vi "UHR-Fleezers Control (fpga) - 10.4.vi"() -> ()   [LabVIEW 2014]
doc: "UHR-Fleezers Instrument Control Code (fpga)"
uses:
  <vilib>/eio/EIONode/EIONode.xnode
  <vilib>/eio/EIOMethodNode/EIOMethodNode.xnode
  <vilib>/rvi/DataTransferAndStorage/Container/XNode/niFpgaContainer.xnode
  <vilib>/Platform/TimedLoop/XDataNode/XDataNode.xnode
  <vilib>/Platform/TimedLoop/XDataNode/nitl_modes.ctl
  <vilib>/Platform/TimedLoop/XDataNode/XDNodeRunTimeDep.lvlib
  <vilib>/Platform/TimedLoop/XDataNode/wakeup.ctl
  <vilib>/Platform/TimedLoop/XDataNode/timing_clust.ctl
  <vilib>/addons/control/pid/fpga.llb/XNode/niFpgaPID.xnode
  <vilib>/rvi/eio/common/nirviEmuTemplateMethod_errors.vi
  <vilib>/rvi/interface/RandomDataEmulation/nirviRandomDataFpgaReadWriteTemplate.vi
panel:
  in  "Connector0/AO6":i16
  in  "Tab Control":T1(tab)=enum."Force FB"
  in  "Trap Pos to FIFO":bool
  in  "AI1 Sets to FIFO":T2={"Set 1"=TRUE, "Set 2"=TRUE, "Set 3"=FALSE}
  in  "N of AI1 Int Acq Sets":i16=2 min=1 max=3 step=1
  out "AI Late Counter":u16
  in  "ai count":u32=400
  out "AI late?":bool
  in  "+ phase":bool
  in  "Phase count adjustment":i16
  out "Relative phase":i16
  in  "AI to FIFO":bool
  out "BD1 Frequency Out 1":u64
  out "BD1 Frequency Out 2":u64
  out "Trap Pos FIFO Timeout":u16
  out "Trap AI FIFO Timeout":u16
  in  "Trap FIFO Set Timeout":i32
  in  "Tab Control 2":T3(tab)
  in  "Swap F1 and F2":bool
  in  "Freq or Amp switch first":bool=TRUE
  in  "Cont. Scan":bool
  in  "Abort scan":bool
  in  "Cycles per step":u64
  in  "Scan BD":bool
  in  "Number of scans":u16
  in  "Scan steps":u64
  in  "Scan freq.  increment":i64
  out "Scanning":bool
  in  "Start scan":bool
  in  "OSK Bd 1":bool
  in  "Reset Bd 1":bool
  in  "RD":bool
  in  "PMODE":bool
  in  "OSK Bd 2":bool
  in  "Reset Bd 2":bool
  in  "Direct RF Box \nCommunication":bool
  in  "Data BD 2":u8 format="%08b"
  in  "Data BD 1":u8 format="%08b"
  in  "Address":u8 format="%02x"
  in  "Update Data":bool
  in  "FPGA Controls\n RF Box":bool
  in  "Number Interlace Cycles":u8=2 min=1 max=3
  in  "Interlace Off Parameters":u8=1 min=1 max=3
  in  "Interlace ON/OFF":bool
  out "DIO Relative phase":i16
  in  "Phase count adjustment (DIO)":i16
  in  "+ phase (DIO)":bool
  out "DIO Late Counter":u16
  out "DIO Late?":bool
  in  "DIO count 1 (ticks)":u32=400
  in  "DIO count 2 (ticks)":u32=400
  in  "DIO count 3 (ticks)":u32=400
  out "AI2 Y Sum Set 2":i16
  out "AI2 Y Sum Set 1":i16
  in  "FB Gains Set 1":T4={"proportional gain (Kc)"=10, "integral gain (Kc*Ts/Ti)"=5, "derivative gain (Kc*Td/Ts)"=0}
  in  "FB Setpoint Set 1":i16 min=0 step=1
  in  "FB Reset Set 1":bool
  in  "FB On/Off Set 1":bool
  in  "FB Reset Set 2":bool
  in  "FB On/Off Set 2":bool
  in  "FB Setpoint Set 2":i16 min=0 step=1
  in  "FB Gains Set 2":T4={"proportional gain (Kc)"=10, "integral gain (Kc*Ts/Ti)"=5, "derivative gain (Kc*Td/Ts)"=0}
  in  "FB output range 2":cluster{"output high":i16, "output low":i16}={"output high"=3000, "output low"=0}
  in  "FB output range 1":cluster{"output high":i16, "output low":i16}={"output high"=3000, "output low"=0}
  out "Scan I":u64
  in  "Amp switch delay":u16=5
  in  "Freq switch delay":u16
  in  "BD 2 Amplitude 1":u16
  in  "BD 1 Amplitude 1":u16
  in  "BD 2 Frequency 1":u64
  in  "BD 1 Frequency 1":u64
  in  "BD 2 Amplitude 2":u16
  in  "BD 1 Amplitude 2":u16
  in  "BD 2 Frequency 2":u64
  in  "BD 1 Frequency 2":u64
  in  "BD 2 Amplitude 3":u16
  in  "BD 1 Amplitude 3":u16
  in  "BD 2 Frequency 3":u64
  in  "BD 1 Frequency 3":u64
  in  "Negate Diff?":bool
  in  "Diff FB Measurement?":bool
  in  "FB Trig Integrate":u32=1
  out "TTrig?":bool
  in  "TTrig Negate Pos":bool=TRUE
  out "Trap Pos FB Int Signal":fxp<+/-,24,9> format="%.18g"
  out "Trap Pos FB Int-Norm Signal":fxp<+/-,16,1> format="%.16g"
  in  "FPGA TTrig Thresh":i64
  in  "FPGA Trap Trig":bool
  out "Trap Pos FB Action":i64
  in  "Trap Pos. FB Offset Factor":i64
  in  "Trap Pos. FB Mult Factor":i64=2
  in  "Trap Pos. FB Range":T5={"output high"=0.999969482421875, "output low"=-1.0}
  in  "Trap Pos. FB Gains":T6={"proportional gain (Kc)"=0.0, "integral gain (Kc*Ts/Ti)"=10.0, "derivative gain (Kc*Td/Ts)"=0.0} {"proportional gain (Kc)" format="%.11g"; "integral gain (Kc*Ts/Ti)" format="%.11g"; "derivative gain (Kc*Td/Ts)" format="%.11g"}
  in  "Trap Pos. FB Reset":bool
  in  "Trap Pos FB Monitor T1 or T2":bool
  in  "AI1 X Scale":u16
  in  "Trap Pos FB Int Count":u16=100
  in  "Trap Pos FB Negate Action":bool
  out "AI1 X Set 2":fxp<+/-,16,1>
  out "AI1 X Set 1":fxp<+/-,16,1>
  in  "Trap Pos. FB SP":fxp<+/-,16,1>
  in  "Force feedback":bool
  out "TTrig Sig":i64
  out "TTrig Fin Thresh":i64
  out "Numeric":i32
  out "AO2 2":i16
  out "AO1 2":i16
  in  "1D or 2D Scan?":bool
  in  "Abort scan (MCL)":bool
  in  "MCL Scan Axis":bool
  in  "Cont. Scan (MCL)":bool
  out "Scan I (MCL)":u64
  in  "Number of scans (MCL)":u16
  out "Scanning MCL":bool
  in  "Scan steps (MCL)":u64
  in  "Cycles per step (MCL)":u64
  in  "Scan freq.  increment (MCL)":i16
  in  "Start scan (MCL)":bool
  in  "AO2":i16
  in  "AO1":i16
  out "MCL Late Counter":u16
  out "MCL Late?":bool
  in  "MCL count":u32=800
  out "MCL Relative Phase":i16
  in  "Phase count adjustment (MCL)":i16
  in  "+ phase (MCL)":bool
  in  "APD Gate Operating Mode":u8 max=2 step=1
  in  "Invert APD Gate":bool
  in  "APD Gate OFF Count":u32=100
  in  "APD Gate ON Count":u32=300
  out "APD 1 Gate Late Counter":u16
  out "APD 1 Gate Late?":bool
  out "APD 1 Gate Relative Phase":i16
  in  "Phase count adjustment (APD 1 Gate)":i16
  in  "+ phase (APD 1 Gate)":bool
  out "APD 2 Counts 0":u32
  out "APD 2 Counts 1":u32
  out "APD 1 Counts 0":u32
  out "APD 1 Counts 1":u32
  out "APD1 out state":bool
  in  "APD 2 AO scale factor":i16=1
  in  "APD 1 AO scale factor":i16=1
  in  "APD to FIFO":bool
  in  "APD Acq Rate Count":u32=20000000
  out "APD Acq Late Counter":u16
  out "APD Acq Late?":bool
  out "APD Acq Relative Phase":i16
  in  "Phase Count Adjustment (APD Acq)":i16
  in  "+ phase (APD Acq)":bool
  in  "Phase count adjustment (APD 2 Gate)":i16
  out "APD 2 Gate Late Counter":u16
  out "APD 2 Gate Late?":bool
  out "APD 2 Gate Relative Phase":i16
  in  "+ phase (APD 2 Gate)":bool
  out "APD2 out state":bool
  in  "Green Filter Flipper":bool
  out "Green FB Signals":T7
  in  "Green FB Count":u32=1200
  out "Green Late Counter":u16
  out "Green FB Late?":bool
  out "Green FB Relative Phase":i16
  in  "Phase count adjustment (Green FB)":i16=10
  in  "+ phase (Green FB)":bool
  out "Green FB Sum":i16
  in  "Green int current ON count adj":u32=150
  in  "Current Out":u16=30000
  in  "Green FB On/Off":bool
  in  "Green FB Setpoint":i16=250 min=0 step=1
  in  "Green FB Gains":T4={"proportional gain (Kc)"=10, "integral gain (Kc*Ts/Ti)"=5, "derivative gain (Kc*Td/Ts)"=0}
  in  "Green FB Reset":bool
  in  "Operating Mode 2":u8=2 max=2 step=1
  in  "Invert GI 2":bool
  in  "Green interlace OFF count 2":u32=900
  in  "Green interlace ON count 2":u32=300
  out "GI Late Counter 2":u16
  out "GI Late? 2":bool
  out "GI Relative phase 2":i16
  in  "Phase count adjustment (GI) 2":i16=20
  in  "+ phase (GI) 2":bool
  in  "Green interlace OFF count":u32=100
  out "GI Relative phase":i16
  in  "Phase count adjustment (GI)":i16
  in  "+ phase (GI)":bool
  out "GI Late?":bool
  in  "Green interlace ON count":u32=300
  out "GI Late Counter":u16
  in  "Invert GI":bool
  in  "Operating Mode":u8 max=2 step=1
  in  "Chassis2/Mod4/AO1":u16
  # "Only one of these can be on\nat a time:"
  # "Raster Scan AOD"
  # "1 (X)"
  # "2 (Y)"
  # "IR Intensity Feedback (RF BD 1)"
  # "FB Triggering Excitation Laser"
  # "AO1 (Y)"
  # "2D"
  # "1D"
  # "AO2 (X)"
  # "APD AO for aligning"
  # "Detection Loop"
  # "Green fluorescent laser digital gate interlacing loop"
  # "0 Forced ON\n1 Forced OFF\n2 Interlacing"
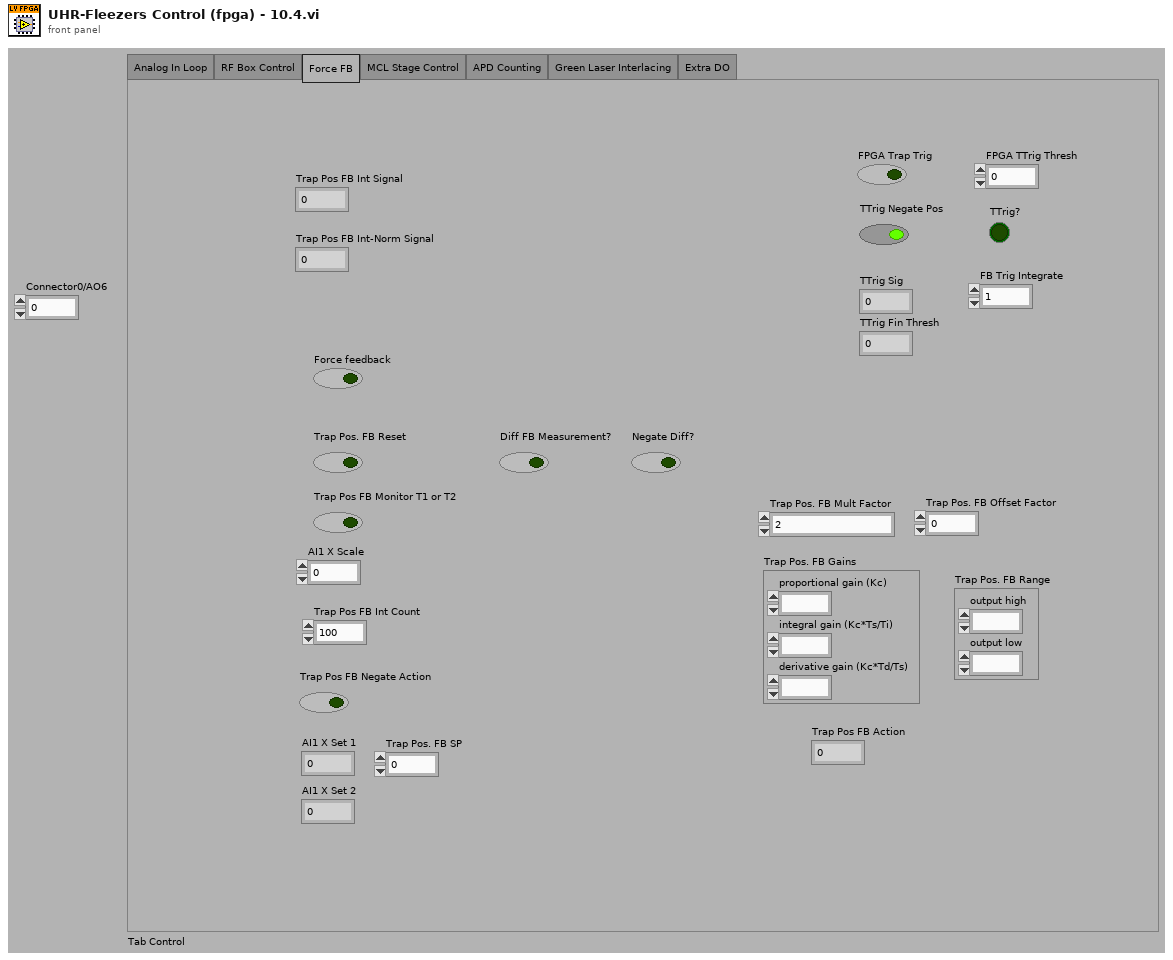
[diagram p1: front panel]
types:
  T1 = enum32{"Analog In Loop", "RF Box Control", "Force FB", "MCL Stage Control", "APD Counting", "Green Laser Interlacing", "Extra DO"}
  T2 = cluster{"Set 1":bool, "Set 2":bool, "Set 3":bool}
  T3 = enum32{"Controls", "Interlacing Frequency and Amplitude Values"}
  T4 = cluster{"proportional gain (Kc)":i16, "integral gain (Kc*Ts/Ti)":i16, "derivative gain (Kc*Td/Ts)":i16}
  T5 = cluster{"output high":fxp<+/-,16,1>, "output low":fxp<+/-,16,1>}
  T6 = cluster{"proportional gain (Kc)":fxp<+/-,16,8>, "integral gain (Kc*Ts/Ti)":fxp<+/-,16,8>, "derivative gain (Kc*Td/Ts)":fxp<+/-,16,8>}
  T7 = cluster{"Green FB Ch 0":i16, "Green FB Ch 1":i16, "Green FB Ch 2":i16}
  T8 = typedef "XDNodeRunTimeDep.lvlib/timing_clust.ctl" = cluster{"Expected End [f-1]":u64, "Actual End [f-1]":u64, "Finished Late? [f-1]":bool, "Expected End [i-1]":u64, "Actual End [i-1]":u64, "Finished Late? [i-1]":bool, "Expected Start [i]":u64, "Actual Start [i]":u64, "Expected Start [f]":u64, "Actual Start [f]":u64, "Source Name":string, "Structure Name":string, "Period":i64, "Deadline":i64, "Offset":i64, "Start":i64, "Priority":i32, "Timeout":i32, "Mode":T9, "Wakeup Reason":T10, "Error":errorcluster, "Source Type":string, "Secondary Source Type":string, "Global End Time":u64, "Global Start Time":u64, "Frame Duration":u64, "Iteration Duration":u64, "Assigned CPU":i32, "I/O Scan Engine Mode":u32}
  T9 = typedef "XDNodeRunTimeDep.lvlib/nitl_modes.ctl" = enum32{"No Change", "Process missed periods, maintain original phase", "Discard missed periods, maintain original phase", "Process missed periods, ignore original phase", "Discard missed periods, ignore original phase"}
  T10 = typedef "XDNodeRunTimeDep.lvlib/wakeup.ctl" = enum32{"Normal", "Aborted", "Asynchronous wakeup", "Timing source error", "Timed loop error", "Timeout"}
  T11 = cluster{"Chassis2/Mod1/AI0":void, "Chassis2/Mod1/AI1":void, "Chassis2/Mod1/AI2":void}
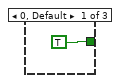
[diagram p2: hidden frame]
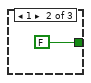
[diagram p3: hidden frame]
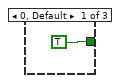
[diagram p5: hidden frame]
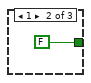
[diagram p6: hidden frame]
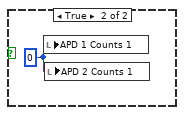
[diagram p7: hidden frame]
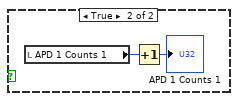
[diagram p9: hidden frame]
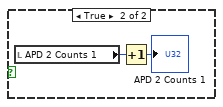
[diagram p10: hidden frame]
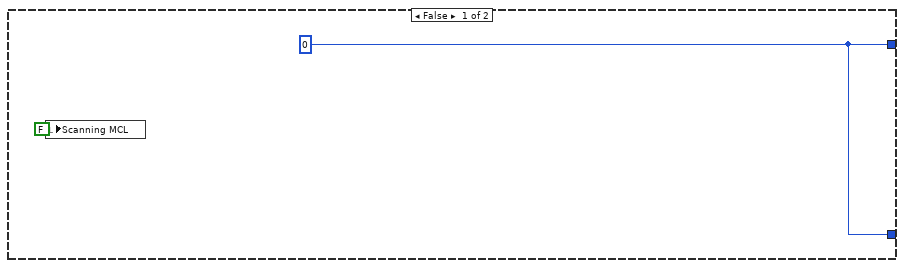
[diagram p11: hidden frame]
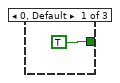
[diagram p12: hidden frame]
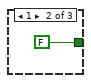
[diagram p13: hidden frame]
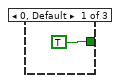
[diagram p14: hidden frame]
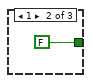
[diagram p15: hidden frame]
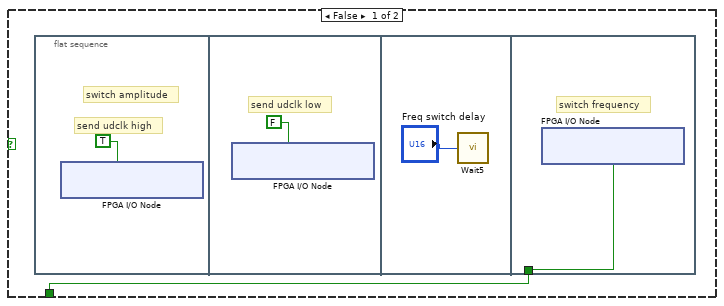
[diagram p18: hidden frame]
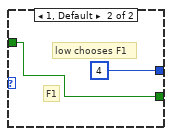
[diagram p20: hidden frame]
diagram:
  w3 = FALSE
  # "timing array current index"
  # "timing array"
  # "timing counter (phase adjusted here)"
  # "late counter"
  n1 = flat-sequence "FPGA initialization to do before running any of the loops" {
    tunnel: [u32 0 ("DIO count 3 (ticks)")] -> w2
    tunnel: [w10] -> _
    frame #0 {
      # "Start up expansion chassis early\nto avoid delays later"
      # "This pin controls udclk on the RF boards.\nWhen initially configuring the boards, this pin needs to be\nconfigured as a high impedance input.  Later it will be switched\nto an output."
      # "Initial setting of DIO data and \naddress to low (before reset).  \nThis needs to happen before the other\ncontrol method loops execute."
      n2 = xnode "FPGA I/O Node"("Chassis2/Mod4/AO0"=u16 0) -> ("Chassis2/Mod1/AI0"=w10)  [unwired: 2 in, 2 out]
      n3 = xnode "FPGA I/O Method Node"("Enable"=FALSE) -> ()  [unwired: 1 in, 1 out]
      n4 = xnode "FPGA I/O Node"("Connector1/DIO0"=FALSE, "Connector1/DIO1"=FALSE, "Connector1/DIO2"=FALSE, "Connector1/DIO3"=FALSE, "Connector1/DIO4"=FALSE, "Connector1/DIO5"=FALSE, "Connector1/DIO6"=FALSE, "Connector1/DIO7"=FALSE, "Connector1/DIO8"=FALSE, "Connector1/DIO9"=FALSE, "Connector1/DIO10"=FALSE, "Connector1/DIO11"=FALSE, "Connector1/DIO12"=FALSE, "Connector1/DIO13"=FALSE, "Connector1/DIO15"=FALSE, "Connector1/DIO20"=FALSE, "Connector1/DIO21"=FALSE, "Connector1/DIO22"=FALSE, "Connector1/DIO23"=FALSE, "Connector1/DIO24"=FALSE, "Connector1/DIO25"=FALSE, "Connector1/DIO26"=FALSE, "Connector1/DIO27"=FALSE, "Connector1/DIO14"=FALSE) -> ()  [unwired: 24 in, 24 out]
    }
  }
  n5 = local read "AO1"() -> (w7:i16)
  n6 = local read "AO2"() -> (w6:i16)
  n7 = node-c288() -> (w5:T8)  [unwired: 1 in]
  n8 = while "APD 1 Counter" {
    tunnel: w2 -> [_]
    stop <- FALSE stop-if-true
    n9 = flat-sequence {
      frame #0 {
        n10 = xnode "FPGA I/O Method Node"("FPGA I/O In"=refnum<k21> "Connector0/DIO0" ("APD 1 DO"), "Timeout"=-1) -> ()  [unwired: 2 out]
      }
      frame #1 {
        n11 = local read "APD1 out state"() -> (w41:bool)
        n12 = case shown="False" w41 {
          frame False {
            n13 = local read "APD 1 Counts 0"() -> (w43:u32)
            n14 = Increment(x=w43) -> (x+1=→"APD 1 Counts 0":u32)
          }
          frame True {
            n15 = local read "APD 1 Counts 1"() -> (w45:u32)
            n16 = Increment(x=w45) -> (x+1=→"APD 1 Counts 1":u32)
          }
        }
      }
    }
  }
  n17 = while "APD 2 Counter" {
    tunnel: w2 -> [_]
    stop <- FALSE stop-if-true
    n18 = flat-sequence {
      frame #0 {
        n19 = xnode "FPGA I/O Method Node"("FPGA I/O In"=refnum<k21> "Connector0/DIO1" ("APD 2 DO"), "Timeout"=-1) -> ()  [unwired: 2 out]
      }
      frame #1 {
        n20 = local read "APD2 out state"() -> (w49:bool)
        n21 = case shown="False" w49 {
          frame False {
            n22 = local read "APD 2 Counts 0"() -> (w51:u32)
            n23 = Increment(x=w51) -> (x+1=→"APD 2 Counts 0":u32)
          }
          frame True {
            n24 = local read "APD 2 Counts 1"() -> (w53:u32)
            n25 = Increment(x=w53) -> (x+1=→"APD 2 Counts 1":u32)
          }
        }
      }
    }
  }
  n26 = while "APD 2 Gating" {
    shift-right: [w57] -> _
    shift-left: w2 -> [w62]
    shift-right: [w56] -> _
    shift-left: w3 -> [w54]
    stop <- FALSE stop-if-true
    n27 = flat-sequence {
      tunnel: w62 -> [w65]
      tunnel: [w66] -> w60
      tunnel: [w65] -> w58
      tunnel: [w64] -> w55
      tunnel: w54 -> [w64]
      tunnel: [w69] -> w61
      tunnel: w60 -> [w69]
      tunnel: [w68] -> w59
      tunnel: w58 -> [w68]
      tunnel: w55 -> [w67]
      tunnel: [w87] -> w57
      tunnel: w61 -> [w98]
      tunnel: w59 -> [w96]
      tunnel: [w91] -> w56
      frame #0 {
        n28 = call "Loop Timer8"("Count(Ticks)"=w65) -> ("Tick Count(Ticks)"=w66:u32)
      }
      frame #1 {
        # "(need 4 channels/APD)"
        n29 = xnode "FPGA I/O Node"("Connector0/DIO8"=w67, "Connector0/DIO9"=w67, "Connector0/DIO10"=w67, "Connector0/DIO11"=w67) -> ()  [unwired: 4 in, 4 out]
      }
      frame #2 {
        n30 = local read "APD Gate ON Count"() -> (w80:u32)
        n31 = local read "APD Gate OFF Count"() -> (w79:u32)
        n32 = feedback #1(TRUE) -> (w93:bool)
        n33 = feedback-in #2(w98) -> ()
        n34 = feedback #2(w98) -> (w81:u32)
        n35 = Not(x=w93) -> (.not. x?=w90:bool)
        n36 = feedback-in #1(w90) -> ()
        n37 = Subtract(x=w98, y=w81) -> (x-y=w97:u32)
        n38 = Select(t=w80, s=w90, f=w79) -> (s? t:f=w95:u32)
        n39 = Subtract(x=w97, y=w96) -> (x-y=w72:u32)
        n40 = Subtract(x=w95, y=w72) -> (x-y=w86:u32)
        n41 = Number To Boolean Array(number=w72) -> (Boolean array=w71:bool[])
        n42 = Or Array Elements(Boolean array=w71) -> (logical OR=w70:bool)
        "APD 2 Gate Late?" <- w70
        n43 = Boolean To (0,1)(Boolean="+ phase (APD 2 Gate)") -> (0, 1=w84:i16)
        n44 = Multiply(x=w84, y="Phase count adjustment (APD 2 Gate)") -> (x*y=w82:i16)
        n45 = Boolean To (0,1)(Boolean=w70) -> (0, 1=w77:i16)
        n46 = Add(x=w86, y=w82) -> (x+y=w87:u32)
        n47 = To Unsigned Word Integer(number=w77) -> (unsigned 16bit integer=w74:u16)
        n48 = feedback #3(i16 0) -> (w89:i16)
        n49 = Subtract(x=w89, y=w82) -> (x-y=w88:i16)
        "APD 2 Gate Relative Phase" <- w88
        n50 = feedback-in #3(w88) -> ()
        n51 = feedback #4(u16 0) -> (w75:u16)
        n52 = Add(x=w74, y=w75) -> (x+y=w73:u16)
        "APD 2 Gate Late Counter" <- w73
        n53 = feedback-in #4(w73) -> ()
        n54 = local read "APD Gate Operating Mode"() -> (w78:u8)
        n55 = case shown="2" w78 {
          tunnel: [TRUE FALSE w104] -> w91
          tunnel: w93 -> [_ _ w102]
          frame 0, Default {
          }
          frame 1 {
          }
          frame 2 {
            n56 = local read "Invert APD Gate"() -> (w101:bool)
            n57 = Not(x=w102) -> (.not. x?=w103:bool)
            n58 = Select(t=w103, s=w101, f=w102) -> (s? t:f=w104:bool)
          }
        }
      }
    }
  }
  n59 = while "DAQ AI set 1" {
    shift-right: [w105] -> _
    shift-left: w2 -> [w110]
    stop <- FALSE stop-if-true
    n60 = flat-sequence {
      tunnel: w110 -> [w120]
      tunnel: [w121] -> w108
      tunnel: [w120] -> w107
      tunnel: [w131] -> w118
      tunnel: [w130] -> w117
      tunnel: [w129] -> w116
      tunnel: [w128] -> w115
      tunnel: [w127] -> w114
      tunnel: [w126] -> w113
      tunnel: [w125] -> w112
      tunnel: [w124] -> w111
      tunnel: [w123] -> w109
      tunnel: w108 -> [w123]
      tunnel: w107 -> [w122]
      tunnel: [w122] -> w106
      tunnel: [w160] -> w105
      tunnel: w118 -> [w188]
      tunnel: w117 -> [w152]
      tunnel: w116 -> [w153]
      tunnel: w115 -> [w187]
      tunnel: w114 -> [w176]
      tunnel: w113 -> [w175]
      tunnel: w112 -> [w174]
      tunnel: w111 -> [w173]
      tunnel: w109 -> [w170]
      tunnel: w106 -> [w167]
      frame #0 {
        n61 = call "Loop Timer3"("Count(Ticks)"=w120) -> ("Tick Count(Ticks)"=w121:u32)
      }
      frame #1 {
        n62 = xnode "FPGA I/O Node"("Connector1/DIO31"=TRUE ("Connector1/DIO33")) -> ("Connector0/AI0"=w131, "Connector0/AI1"=w130, "Connector0/AI2"=w129, "Connector0/AI3"=w128, "Connector0/AI4"=w127, "Connector0/AI5"=w126, "Connector0/AI6"=w125, "Connector0/AI7"=w124)  [unwired: 9 in, 9 out]
      }
      frame #2 {
        w156 = FALSE ("AI to FIFO")
        # "Adjust phase after data acquired if button pressed"
        n63 = feedback #5(i16 1) -> (w180:i16)
        n64 = Increment(x=w180) -> (x+1=w186:i16)
        n65 = Scale By Power Of 2(n="AI1 X Scale", x=w152) -> (x*2^n=w150:dbl)
        n66 = Greater?(x=w186, y="N of AI1 Int Acq Sets") -> (0:w183:bool)
        n67 = Select(t=i16 1, s=w183, f=w186) -> (s? t:f=w185:i16)
        n68 = feedback-in #5(w185) -> ()
        n69 = Divide(x=w150, y=w153) -> (x/y=w149:fxp<+/-,16,1>)
        n70 = feedback #6(w156) -> (w154:bool)
        n71 = feedback #7(w156) -> (w172:bool)
        n72 = case shown="1, Default" w180 {
          tunnel: w153 -> [w210 w218 _]
          tunnel: "AI1 Sets to FIFO" -> [w214 w222 w228]
          tunnel: [w213 w221 w227] -> w177
          tunnel: ["AI to FIFO" w220 w226] -> w171
          tunnel: w172 -> [_ w220 w226]
          tunnel: ["Trap Pos to FIFO" w219 w225] -> w155
          tunnel: w154 -> [_ w219 w225]
          tunnel: w149 -> [w209 w217 _]
          tunnel: [w208 w215 FALSE] -> w136
          tunnel: [w207 w216 u64 0 ("BD1 Frequency Out 2")] -> w135
          frame 1, Default {
            n73 = Unbundle By Name(w214) -> ("Set 1"=w213:bool)
            n74 = local read "BD1 Frequency Out 1"() -> (w207:u64)
            n75 = Compound Arithmetic op=AND("Trap Pos to FIFO", w213, "AI to FIFO") -> (w208:bool)
            "AI2 Y Sum Set 1" <- w210
            "AI1 X Set 1" <- w209
          }
          frame 2 {
            n76 = Unbundle By Name(w222) -> ("Set 2"=w221:bool)
            n77 = local read "BD1 Frequency Out 2"() -> (w216:u64)
            n78 = Compound Arithmetic op=AND(w219, w221, w220) -> (w215:bool)
            "AI2 Y Sum Set 2" <- w218
            "AI1 X Set 2" <- w217
          }
          frame 3 {
            n79 = Unbundle By Name(w228) -> ("Set 3"=w227:bool)
          }
        }
        n80 = And(x=w177, y=w171) -> (x .and. y?=w179:bool)
        n81 = case shown="True" w179 {
          tunnel: w188 -> [_ w242]
          tunnel: w152 -> [_ w241]
          tunnel: w153 -> [_ w240]
          tunnel: w187 -> [_ w239]
          tunnel: w176 -> [_ w238]
          tunnel: w175 -> [_ w237]
          tunnel: w174 -> [_ w236]
          tunnel: w173 -> [_ w235]
          tunnel: 0 ("DMA buffer timeout") -> [_ w244]
          frame False {
          }
          frame True {
            n82 = Build Array(w242, w241, w240, w239, w238, w237, w236, w235) -> (w243:void[])
            n83 = for {
              tunnel: w243 -> [w246] mode=indexing
              tunnel: w244 -> [w247]
              tunnel: [w245] -> w233 mode=indexing
              n84 = xnode ("FIFO Write")("Element"=w246, "Timeout"=w247) -> ("Timed Out?"=w245:bool)  [unwired: 1 in, 1 out]
            }
            n85 = Or Array Elements(Boolean array=w233) -> (logical OR=w230:bool)
            n86 = Boolean To (0,1)(Boolean=w230) -> (0, 1=w232:i16)
            n87 = feedback #8(u16 0) -> (w231:u16)
            n88 = Add(x=w232, y=w231) -> (x+y=w229:u16)
            "Trap AI FIFO Timeout" <- w229
            n89 = feedback-in #8(w229) -> ()
          }
        }
        n90 = feedback-in #6(w155) -> ()
        n91 = feedback-in #7(w171) -> ()
        n92 = case shown="True" w136 {
          tunnel: w135 -> [_ w194]
          tunnel: [u8 0 w191] -> w134
          frame False {
          }
          frame True {
            n93 = Split Number(x=w194) -> (hi(x)=w195:u32, lo(x)=w196:u32)
            n94 = Split Number(x=w195) -> (lo(x)=w197:u16)  [unwired: 1 out]
            n95 = Split Number(x=w196) -> (hi(x)=w198:u16, lo(x)=w199:u16)
            n96 = Build Array "BD 1 nu Stack"(w197, w198, w199) -> (w193:u16[])
            n97 = for {
              tunnel: w193 -> [w206] mode=indexing
              shift-right: [w202] -> w191
              shift-left: u8 0 -> [w203]
              n98 = xnode ("FIFO Method Node")("Element"=w206, "Timeout"="Trap FIFO Set Timeout") -> ("Timed Out?"=w205:bool)  [unwired: 1 in, 1 out]
              n99 = Boolean To (0,1)(Boolean=w205) -> (0, 1=w204:i16)
              n100 = To Unsigned Byte Integer(number=w204) -> (unsigned 8bit integer=w201:u8)
              n101 = Add(x=w201, y=w203) -> (x+y=w202:u8)
            }
          }
        }
        n102 = To Unsigned Word Integer(number=w134) -> (unsigned 16bit integer=w133:u16)
        n103 = feedback #9(u16 0) -> (w147:u16)
        n104 = Add(x=w133, y=w147) -> (x+y=w146:u16)
        "Trap Pos FIFO Timeout" <- w146
        n105 = feedback-in #9(w146) -> ()
        n106 = feedback-in #10(w170) -> ()
        n107 = feedback #10(w170) -> (w169:u32)
        n108 = Subtract(x=w170, y=w169) -> (x-y=w168:u32)
        n109 = xnode "I/O Node"("Connector1/DIO31"=FALSE ("Connector1/DIO34")) -> ()  [unwired: 1 in, 1 out]
        n110 = Subtract(x=w168, y=w167) -> (x-y=w138:u32)
        n111 = Boolean To (0,1)(Boolean="+ phase") -> (0, 1=w163:i16)
        n112 = Multiply(x=w163, y="Phase count adjustment") -> (x*y=w157:i16)
        n113 = Subtract(x="ai count", y=w138) -> (x-y=w161:u32)
        n114 = Number To Boolean Array(number=w138) -> (Boolean array=w139:bool[])
        n115 = feedback #11(i16 0) -> (w159:i16)
        n116 = Add(x=w161, y=w157) -> (x+y=w160:u32)
        n117 = Subtract(x=w159, y=w157) -> (x-y=w158:i16)
        "Relative phase" <- w158
        n118 = feedback-in #11(w158) -> ()
        n119 = Or Array Elements(Boolean array=w139) -> (logical OR=w137:bool)
        "AI late?" <- w137
        n120 = Boolean To (0,1)(Boolean=w137) -> (0, 1=w144:i16)
        n121 = To Unsigned Word Integer(number=w144) -> (unsigned 16bit integer=w141:u16)
        n122 = feedback #12(u16 0) -> (w142:u16)
        n123 = Add(x=w141, y=w142) -> (x+y=w140:u16)
        "AI Late Counter" <- w140
        n124 = feedback-in #12(w140) -> ()
      }
    }
  }
  n125 = while "MCL stage control" {
    shift-right: [w263] -> _
    shift-left: w2 -> [w266]
    shift-right: [w256] -> _
    shift-left: w7 -> [w253]
    shift-right: [w255] -> _
    shift-left: w6 -> [w251]
    i -> [w250]
    stop <- FALSE stop-if-true
    n126 = flat-sequence {
      tunnel: w266 -> [w270]
      tunnel: [w271] -> w262
      tunnel: [w270] -> w260
      tunnel: [w269] -> w254
      tunnel: w253 -> [w269]
      tunnel: [w268] -> w252
      tunnel: w251 -> [w268]
      tunnel: w262 -> [w275]
      tunnel: [w275] -> w261
      tunnel: w260 -> [w274]
      tunnel: [w274] -> w259
      tunnel: w254 -> [w273]
      tunnel: w252 -> [w272]
      tunnel: [w273] -> w249
      tunnel: [w272] -> w248
      tunnel: w261 -> [w285]
      tunnel: w259 -> [w284]
      tunnel: [w285] -> w265
      tunnel: [w284] -> w264
      tunnel: [w283] -> w258
      tunnel: [w282] -> w257
      tunnel: w249 -> [w277]
      tunnel: w248 -> [w276]
      tunnel: [w357] -> w263
      tunnel: w265 -> [w364]
      tunnel: w264 -> [w361]
      tunnel: w258 -> [w359]
      tunnel: w257 -> [w358]
      tunnel: [w359] -> w256
      tunnel: [w358] -> w255
      frame #0 {
        n127 = call "Loop Timer5"("Count(Ticks)"=w270) -> ("Tick Count(Ticks)"=w271:u32)
      }
      frame #1 {
        n128 = xnode "FPGA I/O Node"("Connector0/AO1"=w273, "Connector0/AO2"=w272) -> ()  [unwired: 2 in, 2 out]
      }
      frame #2 {
        n129 = local read "Scanning MCL"() -> (w297:bool)
        n130 = Or(x=w297, y="Start scan (MCL)") -> (x .or. y?=w292:bool)
        n131 = Not(x="Abort scan (MCL)") -> (.not. x?=w290:bool)
        n132 = And(x=w290, y=w292) -> (x .and. y?=w289:bool)
        n133 = case "Raster scan" shown="True" w289 {
          tunnel: [w298 w341] -> w294
          tunnel: "Start scan (MCL)" -> [_ w326]
          tunnel: [w298 w302] -> w278
          frame False {
            w298 = i16 0
            n134 = local write "Scanning MCL"(FALSE ("scanning")) -> ()
          }
          frame True {
            w312 = i16 0
            w311 = u64 0
            # "scan incr."
            # "freq. incr. mult."
            # "count steps"
            # "count number of cycles"
            n135 = feedback #13(w311) -> (w338:u64)
            n136 = Select(t=w311, s=w326, f=w338) -> (s? t:f=w340:u64)
            n137 = Increment(x=w340) -> (x+1=w337:u64)
            n138 = Greater?(x="Cycles per step (MCL)", y=w337) -> (0:w321:bool)
            n139 = Select(t=w337, s=w321, f=w311) -> (s? t:f=w336:u64)
            n140 = feedback-in #13(w336) -> ()
            n141 = feedback #14(w311) -> (w335:u64)
            n142 = Select(t=w311, s=w326, f=w335) -> (s? t:f=w330:u64)
            n143 = Increment(x=w330) -> (x+1=w334:u64)
            n144 = Add(x="Scan steps (MCL)", y="Scan steps (MCL)") -> (x+y=w333:u64)
            n145 = Select(t=w330, s=w321, f=w334) -> (s? t:f=w316:u64)
            n146 = Greater?(x=w333, y=w316) -> (0:w315:bool)
            n147 = Select(t=w316, s=w315, f=w311) -> (s? t:f=w331:u64)
            n148 = feedback-in #14(w331) -> ()
            n149 = Equal?(x="Scan steps (MCL)", y=w316) -> (x = y?=w320:bool)
            n150 = Greater?(x="Scan steps (MCL)", y=w330) -> (0:w329:bool)
            n151 = feedback #15(w312) -> (w332:i16)
            n152 = Select(t=w312, s=w326, f=w332) -> (s? t:f=w318:i16)
            n153 = Increment(x=w318) -> (x+1=w328:i16)
            n154 = Decrement(x=w318) -> (x-1=w327:i16)
            n155 = Select(t=w328, s=w329, f=w327) -> (s? t:f=w319:i16)
            n156 = Select(t=w318, s=w320, f=w319) -> (s? t:f=w317:i16)
            n157 = Select(t=w318, s=w321, f=w317) -> (s? t:f=w313:i16)
            n158 = Select(t=w313, s=w315, f=w312) -> (s? t:f=w314:i16)
            n159 = feedback-in #15(w314) -> ()
            n160 = feedback #16(w311) -> (w325:u64)
            n161 = Select(t=w311, s=w326, f=w325) -> (s? t:f=w300:u64)
            n162 = Increment(x=w300) -> (x+1=w322:u64)
            n163 = Select(t=w300, s=w315, f=w322) -> (s? t:f=w301:u64)
            n164 = Greater?(x="Number of scans (MCL)", y=w301) -> (0:w308:bool)
            n165 = Multiply(x="Scan freq.  increment (MCL)", y=w318) -> (x*y=w341:i16)
            n166 = Select(t=TRUE, s="Cont. Scan (MCL)", f=w308) -> (s? t:f=w307:bool)
            "Scanning MCL" <- w307
            n167 = Select(t=w301, s=w307, f=w311) -> (s? t:f=w323:u64)
            n168 = feedback-in #16(w323) -> ()
            n169 = Increment(x=w301) -> (x+1=→"Scan I (MCL)":u64)
            n170 = To Word Integer(number=w300) -> (16bit integer=w303:i16)
            n171 = Multiply(x=w303, y="Scan freq.  increment (MCL)") -> (x*y=w302:i16)
          }
        }
        n172 = Select(t=w278, s="1D or 2D Scan?", f=i16 0) -> (s? t:f=w279:i16)
        n173 = Select(t=w279, s="MCL Scan Axis", f=w294) -> (s? t:f=w293:i16)
        n174 = Select(t=w294, s="MCL Scan Axis", f=w279) -> (s? t:f=w295:i16)
        n175 = Add(x=w293, y="AO2") -> (x+y=w282:i16)
        n176 = Add(x="AO1", y=w295) -> (x+y=w283:i16)
        "AO1 2" <- w277
        "AO2 2" <- w276
      }
      frame #3 {
        n177 = feedback-in #17(w364) -> ()
        n178 = feedback #17(w364) -> (w363:u32)
        n179 = Boolean To (0,1)(Boolean="+ phase (MCL)") -> (0, 1=w355:i16)
        n180 = Subtract(x=w364, y=w363) -> (x-y=w362:u32)
        n181 = Multiply(x=w355, y="Phase count adjustment (MCL)") -> (x*y=w351:i16)
        n182 = Subtract(x=w362, y=w361) -> (x-y=w343:u32)
        n183 = Subtract(x="MCL count", y=w343) -> (x-y=w353:u32)
        n184 = feedback #18(i16 0) -> (w352:i16)
        n185 = Subtract(x=w352, y=w351) -> (x-y=w350:i16)
        "MCL Relative Phase" <- w350
        n186 = feedback-in #18(w350) -> ()
        n187 = Number To Boolean Array(number=w343) -> (Boolean array=w344:bool[])
        n188 = Or Array Elements(Boolean array=w344) -> (logical OR=w342:bool)
        "MCL Late?" <- w342
        n189 = Boolean To (0,1)(Boolean=w342) -> (0, 1=w349:i16)
        n190 = Add(x=w353, y=w351) -> (x+y=w357:u32)
        n191 = To Unsigned Word Integer(number=w349) -> (unsigned 16bit integer=w346:u16)
        n192 = feedback #19(u16 0) -> (w347:u16)
        n193 = Add(x=w346, y=w347) -> (x+y=w345:u16)
        "MCL Late Counter" <- w345
        n194 = feedback-in #19(w345) -> ()
      }
    }
    "Numeric" <- w250
  }
  n195 = while "APD 1 Gating" {
    shift-right: [w369] -> _
    shift-left: w2 -> [w374]
    shift-right: [w368] -> _
    shift-left: w3 -> [w366]
    stop <- FALSE stop-if-true
    n196 = flat-sequence {
      tunnel: w374 -> [w377]
      tunnel: [w378] -> w372
      tunnel: [w377] -> w370
      tunnel: [w376] -> w367
      tunnel: w366 -> [w376]
      tunnel: [w381] -> w373
      tunnel: w372 -> [w381]
      tunnel: [w380] -> w371
      tunnel: w370 -> [w380]
      tunnel: w367 -> [w379]
      tunnel: [w395] -> w369
      tunnel: w373 -> [w410]
      tunnel: w371 -> [w407]
      tunnel: [w399] -> w368
      frame #0 {
        n197 = call "Loop Timer7"("Count(Ticks)"=w377) -> ("Tick Count(Ticks)"=w378:u32)
      }
      frame #1 {
        # "(need 4 channels/APD)"
        n198 = xnode "FPGA I/O Node"("Connector0/DIO4"=w379, "Connector0/DIO5"=w379, "Connector0/DIO6"=w379, "Connector0/DIO7"=w379) -> ()  [unwired: 4 in, 4 out]
      }
      frame #2 {
        n199 = feedback #20(TRUE) -> (w402:bool)
        n200 = feedback-in #21(w410) -> ()
        n201 = feedback #21(w410) -> (w409:u32)
        n202 = Not(x=w402) -> (.not. x?=w398:bool)
        n203 = feedback-in #20(w398) -> ()
        n204 = Subtract(x=w410, y=w409) -> (x-y=w408:u32)
        n205 = Select(t="APD Gate ON Count", s=w398, f="APD Gate OFF Count") -> (s? t:f=w404:u32)
        n206 = Subtract(x=w408, y=w407) -> (x-y=w383:u32)
        n207 = Subtract(x=w404, y=w383) -> (x-y=w394:u32)
        n208 = Number To Boolean Array(number=w383) -> (Boolean array=w384:bool[])
        n209 = Or Array Elements(Boolean array=w384) -> (logical OR=w382:bool)
        "APD 1 Gate Late?" <- w382
        n210 = Boolean To (0,1)(Boolean="+ phase (APD 1 Gate)") -> (0, 1=w392:i16)
        n211 = Boolean To (0,1)(Boolean=w382) -> (0, 1=w389:i16)
        n212 = Multiply(x=w392, y="Phase count adjustment (APD 1 Gate)") -> (x*y=w390:i16)
        n213 = To Unsigned Word Integer(number=w389) -> (unsigned 16bit integer=w386:u16)
        n214 = Add(x=w394, y=w390) -> (x+y=w395:u32)
        n215 = feedback #22(i16 0) -> (w397:i16)
        n216 = Subtract(x=w397, y=w390) -> (x-y=w396:i16)
        "APD 1 Gate Relative Phase" <- w396
        n217 = feedback-in #22(w396) -> ()
        n218 = feedback #23(u16 0) -> (w387:u16)
        n219 = Add(x=w386, y=w387) -> (x+y=w385:u16)
        "APD 1 Gate Late Counter" <- w385
        n220 = feedback-in #23(w385) -> ()
        n221 = case shown="2" "APD Gate Operating Mode" {
          tunnel: [TRUE FALSE w416] -> w399
          tunnel: w402 -> [_ _ w413]
          frame 0, Default {
          }
          frame 1 {
          }
          frame 2 {
            n222 = Not(x=w413) -> (.not. x?=w415:bool)
            n223 = Select(t=w415, s="Invert APD Gate", f=w413) -> (s? t:f=w416:bool)
          }
        }
      }
    }
  }
  n224 = while "RF box board direct communication loop" {
    tunnel: w2 -> [_]
    stop <- FALSE stop-if-true
    n225 = case "Whether to use direct communication method (only use one method at a time)" shown="True" "Direct RF Box \nCommunication" {
      frame False {
      }
      frame True {
        n226 = case shown="True" "Update Data" {
          frame False {
          }
          frame True {
            n227 = flat-sequence {
              frame #0 {
                n228 = First Call?() -> (First Call?: T/F=w420:bool)
                n229 = case shown="True" w420 {
                  frame False {
                  }
                  frame True {
                    # "If first time data updated, be sure to set WR high\nbefore setting data and address bits."
                    n230 = flat-sequence {
                      frame #0 {
                        n231 = xnode "FPGA I/O Node"("Connector1/DIO15"=TRUE) -> ()  [unwired: 1 in, 1 out]
                      }
                      frame #1 {
                        n232 = call "Wait"("Count(Ticks)"=u8 40 ("DO Delay 3 (Ticks)")) -> ()  [unwired: 1 out]
                      }
                    }
                  }
                }
              }
              frame #1 {
                n233 = Number To Boolean Array(number="Address") -> (Boolean array=w469:bool[])
                n234 = Number To Boolean Array(number="Data BD 1") -> (Boolean array=w470:bool[])
                n235 = Number To Boolean Array(number="Data BD 2") -> (Boolean array=w439:bool[])
                n236 = Index Array(array=w470, index=7) -> (element=w454:bool)
                n237 = Index Array(array=w470, index=6) -> (element=w453:bool)
                n238 = Index Array(array=w470, index=5) -> (element=w452:bool)
                n239 = Index Array(array=w470, index=4) -> (element=w451:bool)
                n240 = Index Array(array=w470, index=3) -> (element=w450:bool)
                n241 = Index Array(array=w470, index=2) -> (element=w449:bool)
                n242 = Index Array(array=w470, index=1) -> (element=w448:bool)
                n243 = Index Array(array=w470, index=0) -> (element=w447:bool)
                n244 = Index Array(array=w469, index=5) -> (element=w446:bool)
                n245 = Index Array(array=w469, index=4) -> (element=w445:bool)
                n246 = Index Array(array=w469, index=3) -> (element=w444:bool)
                n247 = Index Array(array=w469, index=2) -> (element=w443:bool)
                n248 = Index Array(array=w469, index=1) -> (element=w442:bool)
                n249 = Index Array(array=w469, index=0) -> (element=w441:bool)
                n250 = Index Array(array=w439, index=7) -> (element=w430:bool)
                n251 = Index Array(array=w439, index=6) -> (element=w429:bool)
                n252 = Index Array(array=w439, index=5) -> (element=w428:bool)
                n253 = Index Array(array=w439, index=4) -> (element=w427:bool)
                n254 = Index Array(array=w439, index=3) -> (element=w426:bool)
                n255 = Index Array(array=w439, index=2) -> (element=w425:bool)
                n256 = Index Array(array=w439, index=1) -> (element=w424:bool)
                n257 = Index Array(array=w439, index=0) -> (element=w423:bool)
                n258 = xnode "FPGA I/O Node"("Connector1/DIO0"=w454, "Connector1/DIO1"=w453, "Connector1/DIO2"=w452, "Connector1/DIO3"=w451, "Connector1/DIO4"=w450, "Connector1/DIO5"=w449, "Connector1/DIO6"=w448, "Connector1/DIO7"=w447, "Connector1/DIO8"=w446, "Connector1/DIO9"=w445, "Connector1/DIO10"=w444, "Connector1/DIO11"=w443, "Connector1/DIO12"=w442, "Connector1/DIO13"=w441, "Connector1/DIO20"=w430, "Connector1/DIO21"=w429, "Connector1/DIO22"=w428, "Connector1/DIO23"=w427, "Connector1/DIO24"=w426, "Connector1/DIO25"=w425, "Connector1/DIO26"=w424, "Connector1/DIO27"=w423) -> ()  [unwired: 22 in, 22 out]
              }
              frame #2 {
                # "wait and then apply write signal"
                n259 = call "Wait2"("Count(Ticks)"=u8 40 ("DO Delay 1 (Ticks)")) -> ()  [unwired: 1 out]
              }
              frame #3 {
                # "sending bit low writes data to board buffer"
                n260 = xnode "FPGA I/O Node"("Connector1/DIO15"=FALSE) -> ()  [unwired: 1 in, 1 out]
              }
              frame #4 {
                # "wait then return write signal"
                n261 = call "Wait3"("Count(Ticks)"=u8 40 ("DO Delay 2 (Ticks)")) -> ()  [unwired: 1 out]
              }
              frame #5 {
                # "sending bit high makes ready to\nwrite more data"
                n262 = xnode "FPGA I/O Node"("Connector1/DIO15"=TRUE) -> ()  [unwired: 1 in, 1 out]
              }
            }
          }
        }
      }
    }
  }
  n263 = while "Control APD data integration - stream to host" {
    shift-right: [w479] -> _
    shift-left: w2 -> [w484]
    stop <- FALSE stop-if-true
    n264 = flat-sequence {
      tunnel: w484 -> [w486]
      tunnel: [w487] -> w482
      tunnel: [w486] -> w480
      tunnel: [w495] -> w483
      tunnel: w482 -> [w495]
      tunnel: [w494] -> w481
      tunnel: w480 -> [w494]
      tunnel: [w493] -> w478
      tunnel: [w492] -> w477
      tunnel: [w529] -> w479
      tunnel: w483 -> [w541]
      tunnel: w481 -> [w538]
      tunnel: w478 -> [w522]
      tunnel: w477 -> [w521]
      frame #0 {
        n265 = call "Loop Timer6"("Count(Ticks)"=w486) -> ("Tick Count(Ticks)"=w487:u32)
      }
      frame #1 {
        n266 = flat-sequence {
          tunnel: [w497] -> w491
          tunnel: w491 -> [w499]
          tunnel: [w501] -> w490
          tunnel: [w500] -> w489
          tunnel: [w499] -> w488
          tunnel: [w507] -> w492
          tunnel: [w508] -> w493
          tunnel: w490 -> [w508]
          tunnel: w489 -> [w507]
          tunnel: w488 -> [w506]
          frame #0 {
            # "use two separate variable so each APD won't\nhave to wait to read"
            n267 = feedback #24(FALSE) -> (w496:bool)
            "APD1 out state" <- w496
            "APD2 out state" <- w496
            n268 = Not(x=w496) -> (.not. x?=w497:bool)
            n269 = feedback-in #24(w497) -> ()
          }
          frame #1 {
            n270 = local read "APD 1 Counts 1"() -> (w505:u32)
            n271 = local read "APD 1 Counts 0"() -> (w504:u32)
            n272 = local read "APD 2 Counts 1"() -> (w503:u32)
            n273 = local read "APD 2 Counts 0"() -> (w502:u32)
            n274 = Select(t=w505, s=w499, f=w504) -> (s? t:f=w501:u32)
            n275 = Select(t=w503, s=w499, f=w502) -> (s? t:f=w500:u32)
          }
          frame #2 {
            n276 = case shown="False" w506 {
              frame False {
                w509 = u32 0 ("APD 1 Counts 0")
                n277 = local write "APD 1 Counts 0"(w509) -> ()
                n278 = local write "APD 2 Counts 0"(w509) -> ()
              }
              frame True {
                w510 = u32 0 ("APD 1 Counts 1")
                n279 = local write "APD 1 Counts 1"(w510) -> ()
                n280 = local write "APD 2 Counts 1"(w510) -> ()
              }
            }
          }
        }
      }
      frame #2 {
        n281 = feedback-in #25(w541) -> ()
        n282 = feedback #25(w541) -> (w540:u32)
        n283 = Subtract(x=w541, y=w540) -> (x-y=w539:u32)
        n284 = Subtract(x=w539, y=w538) -> (x-y=w514:u32)
        n285 = case shown="True" "APD to FIFO" {
          tunnel: w522 -> [_ w544]
          tunnel: w521 -> [_ w542]
          frame False {
          }
          frame True {
            n286 = flat-sequence {
              tunnel: 0 ("Timeout") -> [w546]
              tunnel: w544 -> [w547]
              tunnel: [w546] -> w543
              tunnel: w543 -> [w549]
              tunnel: w542 -> [w548]
              frame #0 {
                n287 = xnode ("FIFO Write")("Element"=w547, "Timeout"=w546) -> ()  [unwired: 1 in, 2 out]
              }
              frame #1 {
                n288 = xnode ("FIFO Write")("Element"=w548, "Timeout"=w549) -> ()  [unwired: 1 in, 2 out]
              }
            }
          }
        }
        n289 = Subtract(x="APD Acq Rate Count", y=w514) -> (x-y=w530:u32)
        n290 = Number To Boolean Array(number=w514) -> (Boolean array=w515:bool[])
        n291 = Or Array Elements(Boolean array=w515) -> (logical OR=w513:bool)
        "APD Acq Late?" <- w513
        n292 = Boolean To (0,1)(Boolean=w513) -> (0, 1=w520:i16)
        n293 = To Unsigned Word Integer(number=w520) -> (unsigned 16bit integer=w517:u16)
        n294 = Boolean To (0,1)(Boolean="+ phase (APD Acq)") -> (0, 1=w526:i16)
        n295 = feedback #26(u16 0) -> (w518:u16)
        n296 = Add(x=w517, y=w518) -> (x+y=w516:u16)
        "APD Acq Late Counter" <- w516
        n297 = feedback-in #26(w516) -> ()
        n298 = Multiply(x=w526, y="Phase Count Adjustment (APD Acq)") -> (x*y=w523:i16)
        n299 = Add(x=w530, y=w523) -> (x+y=w529:u32)
        n300 = feedback #27(i16 0) -> (w528:i16)
        n301 = Subtract(x=w528, y=w523) -> (x-y=w525:i16)
        "APD Acq Relative Phase" <- w525
        n302 = feedback-in #27(w525) -> ()
        n303 = To Word Integer(number=w522) -> (16bit integer=w531:i16)
        n304 = To Word Integer(number=w521) -> (16bit integer=w532:i16)
        n305 = Multiply(x="APD 1 AO scale factor", y=w531) -> (x*y=w512:i16)
        n306 = Multiply(x="APD 2 AO scale factor", y=w532) -> (x*y=w511:i16)
        n307 = xnode "FPGA I/O Node"("Connector0/AO5"=w512, "Connector0/AO7"=w511) -> ()  [unwired: 2 in, 2 out]
      }
    }
  }
  n308 = timed-loop "RF box board DIO control: control bits" {
    timing: w5 -> [_]
    timing-out: [_] -> w4
    tunnel: [w550] -> _
    tunnel: w2 -> [w550]
    stop <- FALSE stop-if-true
    n309 = xnode "FPGA I/O Node"("Connector1/DIO16"="RD", "Connector1/DIO17"="PMODE", "Connector1/DIO18"="OSK Bd 1", "Connector1/DIO19"="Reset Bd 1", "Connector1/DIO28"="OSK Bd 2", "Connector1/DIO29"="Reset Bd 2") -> ()  [unwired: 6 in, 6 out]
  }
  n310 = while "Green fluorescent laser interlacing (DO to IA 532 nm AOM ME amp)." {
    shift-right: [w563] -> _
    shift-left: w2 -> [w568]
    shift-right: [w562] -> _
    shift-left: FALSE -> [w560]
    stop <- FALSE stop-if-true
    n311 = flat-sequence {
      tunnel: w568 -> [w571]
      tunnel: [w572] -> w566
      tunnel: [w571] -> w564
      tunnel: [w570] -> w561
      tunnel: w560 -> [w570]
      tunnel: [w575] -> w567
      tunnel: w566 -> [w575]
      tunnel: [w574] -> w565
      tunnel: w564 -> [w574]
      tunnel: w561 -> [w573]
      tunnel: [w584] -> w563
      tunnel: w567 -> [w604]
      tunnel: w565 -> [w601]
      tunnel: [w593] -> w562
      frame #0 {
        n312 = call "Loop Timer4"("Count(Ticks)"=w571) -> ("Tick Count(Ticks)"=w572:u32)
      }
      frame #1 {
        n313 = xnode "FPGA I/O Node"("Connector1/DIO37"=w573, "Connector1/DIO38"=w573, "Connector1/DIO39"=w573) -> ()  [unwired: 3 in, 3 out]
      }
      frame #2 {
        n314 = feedback-in #28(w604) -> ()
        n315 = feedback #28(w604) -> (w603:u32)
        n316 = Subtract(x=w604, y=w603) -> (x-y=w602:u32)
        n317 = Subtract(x=w602, y=w601) -> (x-y=w577:u32)
        n318 = Number To Boolean Array(number=w577) -> (Boolean array=w578:bool[])
        n319 = Or Array Elements(Boolean array=w578) -> (logical OR=w576:bool)
        "GI Late?" <- w576
        n320 = Boolean To (0,1)(Boolean="+ phase (GI)") -> (0, 1=w589:i16)
        n321 = Multiply(x=w589, y="Phase count adjustment (GI)") -> (x*y=w586:i16)
        n322 = Boolean To (0,1)(Boolean=w576) -> (0, 1=w583:i16)
        n323 = To Unsigned Word Integer(number=w583) -> (unsigned 16bit integer=w580:u16)
        n324 = feedback #29(i16 0) -> (w587:i16)
        n325 = feedback #30(u16 0) -> (w581:u16)
        n326 = Add(x=w580, y=w581) -> (x+y=w579:u16)
        "GI Late Counter" <- w579
        n327 = feedback-in #30(w579) -> ()
        n328 = Subtract(x=w587, y=w586) -> (x-y=w585:i16)
        "GI Relative phase" <- w585
        n329 = feedback-in #29(w585) -> ()
        n330 = feedback #31(TRUE) -> (w596:bool)
        n331 = case shown="2" "Operating Mode" {
          tunnel: [TRUE FALSE w610] -> w593
          tunnel: w596 -> [_ _ w607]
          frame 0, Default {
          }
          frame 1 {
          }
          frame 2 {
            n332 = Not(x=w607) -> (.not. x?=w609:bool)
            n333 = Select(t=w609, s="Invert GI", f=w607) -> (s? t:f=w610:bool)
          }
        }
        n334 = Not(x=w596) -> (.not. x?=w592:bool)
        n335 = Select(t="Green interlace ON count", s=w592, f="Green interlace OFF count") -> (s? t:f=w598:u32)
        n336 = Subtract(x=w598, y=w577) -> (x-y=w590:u32)
        n337 = Add(x=w590, y=w586) -> (x+y=w584:u32)
        n338 = feedback-in #31(w592) -> ()
      }
    }
  }
  n339 = while "Green fluorescent laser interlacing (Current to IA 532 nm AOM ME amp)." {
    shift-right: [w616] -> _
    shift-left: w2 -> [w619]
    shift-right: [w613] -> _
    shift-left: u16 0 -> [w611]
    stop <- FALSE stop-if-true
    n340 = flat-sequence {
      tunnel: w619 -> [w622]
      tunnel: [w623] -> w618
      tunnel: [w622] -> w617
      tunnel: [w621] -> w612
      tunnel: w611 -> [w621]
      tunnel: [w626] -> w615
      tunnel: w618 -> [w626]
      tunnel: [w625] -> w614
      tunnel: w617 -> [w625]
      tunnel: w612 -> [w624]
      tunnel: [w635] -> w616
      tunnel: [w652] -> w613
      tunnel: w615 -> [w665]
      tunnel: w614 -> [w662]
      frame #0 {
        n341 = call "Loop Timer10"("Count(Ticks)"=w622) -> ("Tick Count(Ticks)"=w623:u32)
      }
      frame #1 {
        n342 = xnode "FPGA I/O Node"("Chassis2/Mod4/AO0"=w624) -> ()  [unwired: 1 in, 1 out]
      }
      frame #2 {
        n343 = Subtract(x="Green interlace OFF count 2", y="Green int current ON count adj") -> (x-y=w644:u32)
        n344 = feedback-in #32(w665) -> ()
        n345 = feedback #32(w665) -> (w664:u32)
        n346 = Add(x="Green int current ON count adj", y="Green interlace ON count 2") -> (x+y=w645:u32)
        n347 = Subtract(x=w665, y=w664) -> (x-y=w663:u32)
        n348 = Subtract(x=w663, y=w662) -> (x-y=w628:u32)
        n349 = Number To Boolean Array(number=w628) -> (Boolean array=w629:bool[])
        n350 = Boolean To (0,1)(Boolean="+ phase (GI) 2") -> (0, 1=w641:i16)
        n351 = Or Array Elements(Boolean array=w629) -> (logical OR=w627:bool)
        "GI Late? 2" <- w627
        n352 = Boolean To (0,1)(Boolean=w627) -> (0, 1=w634:i16)
        n353 = Multiply(x=w641, y="Phase count adjustment (GI) 2") -> (x*y=w637:i16)
        n354 = To Unsigned Word Integer(number=w634) -> (unsigned 16bit integer=w630:u16)
        n355 = feedback #33(u16 0) -> (w632:u16)
        n356 = Add(x=w630, y=w632) -> (x+y=w631:u16)
        "GI Late Counter 2" <- w631
        n357 = feedback-in #33(w631) -> ()
        n358 = feedback #34(i16 0) -> (w638:i16)
        n359 = Subtract(x=w638, y=w637) -> (x-y=w636:i16)
        "GI Relative phase 2" <- w636
        n360 = feedback-in #34(w636) -> ()
        n361 = feedback #35(TRUE) -> (w657:bool)
        n362 = case shown="2" "Operating Mode 2" {
          tunnel: [TRUE FALSE w682] -> w646
          tunnel: w657 -> [_ _ w679]
          frame 0, Default {
          }
          frame 1 {
          }
          frame 2 {
            n363 = Not(x=w679) -> (.not. x?=w681:bool)
            n364 = Select(t=w681, s="Invert GI 2", f=w679) -> (s? t:f=w682:bool)
          }
        }
        n365 = And(x=w646, y="Green FB On/Off") -> (x .and. y?=w647:bool)
        n366 = case shown="True" w647 {
          tunnel: "Current Out" -> [w666 _]
          tunnel: [w666 w671] -> w651
          frame False {
          }
          frame True {
            n367 = local read "Green FB Sum"() -> (w667:i16)
            n368 = call "Slower PID.vi"("process variable"=w667, "reset?"="Green FB Reset", "setpoint"="Green FB Setpoint", "PID gains (x 2^8)"="Green FB Gains", "output range"=cluster{"output high":i16, "output low":i16} {"output high"=32767, "output low"=-32768} ("Green FB output range")) -> ("output"=w675:i16)  [unwired: 10 out]
            n369 = To Long Integer(number=w675) -> (32bit integer=w668:i32)
            n370 = Add(x=w668, y=32768) -> (x+y=w670:i32)
            n371 = To Unsigned Word Integer(number=w670) -> (unsigned 16bit integer=w671:u16)
          }
        }
        n372 = Not(x=w657) -> (.not. x?=w654:bool)
        n373 = Select(t=w645, s=w654, f=w644) -> (s? t:f=w659:u32)
        n374 = Subtract(x=w659, y=w628) -> (x-y=w639:u32)
        n375 = Add(x=w639, y=w637) -> (x+y=w635:u32)
        n376 = feedback-in #35(w654) -> ()
        n377 = Boolean To (0,1)(Boolean=w646) -> (0, 1=w653:i16)
        n378 = To Unsigned Word Integer(number=w653) -> (unsigned 16bit integer=w650:u16)
        n379 = Multiply(x=w650, y=w651) -> (x*y=w652:u16)
      }
    }
  }
  n380 = while "Green excitation laser feedback measurement" {
    shift-right: [w683] -> _
    shift-left: w2 -> [w688]
    stop <- FALSE stop-if-true
    n381 = flat-sequence {
      tunnel: w688 -> [w690]
      tunnel: [w691] -> w686
      tunnel: [w690] -> w684
      tunnel: [w698] -> w687
      tunnel: w686 -> [w698]
      tunnel: [w697] -> w685
      tunnel: w684 -> [w697]
      tunnel: [w710] -> w683
      tunnel: w687 -> [w721]
      tunnel: w685 -> [w718]
      frame #0 {
        n382 = call "Loop Timer9"("Count(Ticks)"=w690) -> ("Tick Count(Ticks)"=w691:u32)
      }
      frame #1 {
        n383 = xnode "FPGA I/O Node"("Connector1/DIO35"=TRUE) -> ("Chassis2/Mod1/AI0"=w696, "Chassis2/Mod1/AI1"=w695, "Chassis2/Mod1/AI2"=w692)  [unwired: 4 in, 4 out]
        "Green FB Sum" <- w692
        n384 = Bundle("Chassis2/Mod1/AI0"=w696, "Chassis2/Mod1/AI1"=w695, "Chassis2/Mod1/AI2"=w692) -> (→"Green FB Signals":T11)  [unwired: 1 out]
      }
      frame #2 {
        n385 = feedback-in #36(w721) -> ()
        n386 = feedback #36(w721) -> (w720:u32)
        n387 = Subtract(x=w721, y=w720) -> (x-y=w719:u32)
        n388 = xnode "FPGA I/O Node"("Connector1/DIO35"=FALSE) -> ()  [unwired: 1 in, 1 out]
        n389 = Subtract(x=w719, y=w718) -> (x-y=w700:u32)
        n390 = Subtract(x="Green FB Count", y=w700) -> (x-y=w714:u32)
        n391 = Number To Boolean Array(number=w700) -> (Boolean array=w701:bool[])
        n392 = Or Array Elements(Boolean array=w701) -> (logical OR=w699:bool)
        "Green FB Late?" <- w699
        n393 = Boolean To (0,1)(Boolean="+ phase (Green FB)") -> (0, 1=w712:i16)
        n394 = Boolean To (0,1)(Boolean=w699) -> (0, 1=w706:i16)
        n395 = Multiply(x=w712, y="Phase count adjustment (Green FB)") -> (x*y=w707:i16)
        n396 = Add(x=w714, y=w707) -> (x+y=w710:u32)
        n397 = To Unsigned Word Integer(number=w706) -> (unsigned 16bit integer=w703:u16)
        n398 = feedback #37(i16 0) -> (w709:i16)
        n399 = Subtract(x=w709, y=w707) -> (x-y=w708:i16)
        "Green FB Relative Phase" <- w708
        n400 = feedback-in #37(w708) -> ()
        n401 = feedback #38(u16 0) -> (w704:u16)
        n402 = Add(x=w703, y=w704) -> (x+y=w702:u16)
        "Green Late Counter" <- w702
        n403 = feedback-in #38(w702) -> ()
      }
    }
  }
  n404 = while "Control Additional IO (Green laser flip mount)" {
    stop <- FALSE stop-if-true
    n405 = xnode "FPGA I/O Node"("Connector0/DIO3"="Green Filter Flipper", "Chassis2/Mod4/AO1"="Chassis2/Mod4/AO1", "Connector0/AO6"="Connector0/AO6") -> ()  [unwired: 3 in, 3 out]
    n406 = call "Loop Timer2"("Count(Ticks)"=u32 40000 ("Extra DO Counts")) -> ()  [unwired: 1 out]
  }
  n407 = while "RF box board DIO control: parallel communication" {
    shift-right: [w733] -> _
    shift-left: w2 -> [w732]
    shift-right: [w731] -> _
    shift-left: FALSE ("Swap F1 and F2") -> [w730]
    stop <- FALSE stop-if-true
    n408 = flat-sequence {
      tunnel: w730 -> [w737]
      tunnel: w732 -> [w735]
      tunnel: [w737] -> w729
      tunnel: [w736] -> w728
      tunnel: [w735] -> w727
      tunnel: [w743] -> w733
      tunnel: [w742] -> w731
      tunnel: w729 -> [w741]
      tunnel: w728 -> [w739]
      tunnel: w727 -> [w738]
      frame #0 {
        n409 = call "Loop Timer"("Count(Ticks)"=w735) -> ("Tick Count(Ticks)"=w736:u32)
      }
      frame #1 {
        n410 = flat-sequence {
          tunnel: ["FPGA Controls\n RF Box"] -> w740
          tunnel: w741 -> [w744]
          tunnel: [w784] -> w743
          tunnel: [w797] -> w742
          tunnel: w740 -> [w796]
          tunnel: w739 -> [w790]
          tunnel: w738 -> [w787]
          frame #0 {
            n411 = case shown="True" "FPGA Controls\n RF Box" {
              tunnel: w744 -> [_ w746]
              frame False {
              }
              frame True {
                n412 = flat-sequence {
                  tunnel: w746 -> [w752]
                  frame #0 {
                    n413 = First Call?() -> (First Call?: T/F=w747:bool)
                    n414 = case shown="True" w747 {
                      frame False {
                      }
                      frame True {
                        # "If first time data updated, be sure to set WR high and UDCLK low\nbefore setting data and address bits."
                        n415 = xnode "FPGA I/O Method Node"("Enable"=TRUE) -> ("FPGA I/O Out"=w749:refnum<k21>)  [unwired: 1 in]
                        n416 = xnode "FPGA I/O Node"("Connector1/DIO15"=TRUE) -> ()  [unwired: 1 in, 1 out]
                        n417 = xnode "FPGA I/O Node"("I/O Item"=FALSE ("Connector1/DIO30"), "FPGA I/O In"=w749) -> ()  [unwired: 1 out]
                      }
                    }
                  }
                  frame #1 {
                    n418 = case shown="True" "Freq or Amp switch first" {
                      tunnel: w752 -> [w754 w759]
                      frame False {
                        n419 = flat-sequence {
                          tunnel: w754 -> [w758]
                          frame #0 {
                            # "switch amplitude"
                            # "send udclk high"
                            n420 = xnode "FPGA I/O Node"("Connector1/DIO30"=TRUE ("Connector1/DIO15")) -> ()  [unwired: 1 in, 1 out]
                          }
                          frame #1 {
                            # "send udclk low"
                            n421 = xnode "FPGA I/O Node"("Connector1/DIO30"=FALSE ("Connector1/DIO15")) -> ()  [unwired: 1 in, 1 out]
                          }
                          frame #2 {
                            n422 = call "Wait5"("Count(Ticks)"="Freq switch delay") -> ()  [unwired: 1 out]
                          }
                          frame #3 {
                            # "switch frequency"
                            n423 = xnode "FPGA I/O Node"("Connector1/DIO36"=w758) -> ()  [unwired: 1 in, 1 out]
                          }
                        }
                      }
                      frame True {
                        n424 = flat-sequence {
                          tunnel: w759 -> [w760]
                          frame #0 {
                            # "switch frequency"
                            n425 = xnode "FPGA I/O Node"("Connector1/DIO36"=w760) -> ()  [unwired: 1 in, 1 out]
                          }
                          frame #1 {
                            n426 = call "Wait4"("Count(Ticks)"="Amp switch delay") -> ()  [unwired: 1 out]
                          }
                          frame #2 {
                            # "switch amplitude"
                            # "send udclk high"
                            n427 = xnode "FPGA I/O Node"("Connector1/DIO30"=TRUE ("Connector1/DIO15")) -> ()  [unwired: 1 in, 1 out]
                          }
                          frame #3 {
                            # "send udclk low"
                            n428 = xnode "FPGA I/O Node"("Connector1/DIO30"=FALSE ("Connector1/DIO15")) -> ()  [unwired: 1 in, 1 out]
                          }
                        }
                      }
                    }
                  }
                }
              }
            }
          }
          frame #1 {
            # "This is the prior cycle's on time"
            # "increment timing\nindex, reset to 0 if \nend of matrix"
            # "Reset to begginning (1) when number of cycles reached."
            # "timing index"
            # "build byte stacks for writing data\n(must correspond to addresses array constant)"
            # "Timing housekeeping"
            # "Adjust phase if late\n(maintains constant phase relationship between cycles)"
            n429 = feedback #39(u8 0 ("t")) -> (w793:u8)
            n430 = Increment(x=w793) -> (x+1=w837:u8)
            n431 = Increment(x="Number Interlace Cycles") -> (x+1=w832:u8)
            n432 = Equal?(x=w837, y=w832) -> (x = y?=w839:bool)
            n433 = Select(t=u8 1, s=w839, f=w837) -> (s? t:f=w792:u8)
            n434 = feedback-in #39(w792) -> ()
            n435 = Increment(x=w792) -> (x+1=w834:u8)
            n436 = Equal?(x=w834, y=w832) -> (x = y?=w835:bool)
            n437 = Select(t=u8 1, s=w835, f=w834) -> (s? t:f=w831:u8)
            n438 = Select(t=w831, s="Interlace ON/OFF", f="Interlace Off Parameters") -> (s? t:f=w815:u8)
            n439 = case shown="1, Default" w815 {
              tunnel: [w888 "BD 1 Frequency 2" "BD 1 Frequency 3"] -> w827
              tunnel: [w887 "BD 2 Frequency 2" "BD 2 Frequency 3"] -> w816
              tunnel: ["BD 2 Amplitude 1" "BD 2 Amplitude 2" "BD 2 Amplitude 3"] -> w772
              tunnel: [w876 w1054 "BD 1 Amplitude 3"] -> w775
              frame 1, Default {
                w883 = u64 0 ("f")
                # "Trap 1"
                n440 = local read "Scanning"() -> (w889:bool)
                n441 = case "For position feedback" shown="True" "Force feedback" {
                  tunnel: [i64 0 w907] -> w873
                  frame False {
                  }
                  frame True {
                    w899 = fxp<+/-,24,9> 0.0 ("AI1 X Set 2")
                    w910 = u16 0
                    n442 = local read "AI1 X Set 1"() -> (w903:fxp<+/-,16,1>)
                    n443 = local read "AI1 X Set 2"() -> (w904:fxp<+/-,16,1>)
                    n444 = case shown="False" "Diff FB Measurement?" {
                      tunnel: w904 -> [w915 w924]
                      tunnel: w903 -> [w914 w925]
                      tunnel: [w912 w916] -> w901
                      frame False {
                        n445 = Select(t=w914, s="Trap Pos FB Monitor T1 or T2", f=w915) -> (s? t:f=w912:fxp<+/-,16,1>)
                      }
                      frame True {
                        n446 = Subtract(x=w925, y=w924) -> (x-y=w917:fxp<+/-,17,2>)
                        n447 = Not(x="Negate Diff?") -> (.not. x?=w923:bool)
                        n448 = Boolean To (0,1)(Boolean="Negate Diff?") -> (0, 1=w921:i16)
                        n449 = Boolean To (0,1)(Boolean=w923) -> (0, 1=w922:i16)
                        n450 = Negate(x=w921) -> (-x=w920:i16)
                        n451 = Add(x=w920, y=w922) -> (x+y=w918:i16)
                        n452 = Multiply(x=w918, y=w917) -> (x*y=w916:fxp<+/-,32,17>)
                      }
                    }
                    n453 = feedback #40(w910) -> (w911:u16)
                    n454 = Increment(x=w911) -> (x+1=w909:u16)
                    n455 = Greater Or Equal?(x=w909, y="Trap Pos FB Int Count") -> (x >= y?=w902:bool)
                    n456 = Select(t=w910, s=w902, f=w909) -> (s? t:f=w908:u16)
                    n457 = feedback-in #40(w908) -> ()
                    n458 = feedback #41(w899) -> (w900:fxp<+/-,24,9>)
                    n459 = Add(x=w901, y=w900) -> (x+y=w896:fxp<+/-,24,9>)
                    n460 = Select(t=w899, s=w902, f=w896) -> (s? t:f=w898:fxp<+/-,24,9>)
                    n461 = feedback-in #41(w898) -> ()
                    n462 = feedback #42(i64 0) -> (w906:i64)
                    n463 = case shown="True" w902 {
                      tunnel: [w926 w932] -> w907
                      tunnel: w906 -> [w926 _]
                      tunnel: "Trap Pos FB Int Count" -> [_ w941]
                      tunnel: w896 -> [_ w942]
                      frame False {
                      }
                      frame True {
                        w936 = u32 0
                        n464 = Divide(x=w942, y=w941) -> (x/y=w940:fxp<+/-,16,1>)
                        "Trap Pos FB Int-Norm Signal" <- w940
                        n465 = xnode ("PID")("process variable"=w940, "reset?"="Trap Pos. FB Reset", "setpoint"="Trap Pos. FB SP", "PID gains"="Trap Pos. FB Gains", "output range"="Trap Pos. FB Range") -> ("output"=w951:fxp<+/-,16,1>)
                        n466 = Negate(x=w951) -> (-x=w950:fxp<+/-,17,2>)
                        n467 = Select(t=w950, s="Trap Pos FB Negate Action", f=w951) -> (s? t:f=w947:fxp<+/-,17,2>)
                        n468 = Scale By Power Of 2(n=u32 15, x=u32 1) -> (x*2^n=w944:u32)
                        n469 = Multiply(x=w947, y=w944) -> (x*y=w943:fxp<+/-,17,17>)
                        n470 = To Quad Integer(1:w943) -> (0:w955:i64)
                        "Trap Pos FB Action" <- w955
                        n471 = Multiply(x=w955, y="Trap Pos. FB Mult Factor") -> (x*y=w953:i64)
                        n472 = Add(x=w953, y="Trap Pos. FB Offset Factor") -> (x+y=w932:i64)
                        n473 = feedback #43(w936) -> (w938:u32)
                        n474 = Increment(x=w938) -> (x+1=w927:u32)
                        n475 = Greater Or Equal?(x=w927, y="FB Trig Integrate") -> (x >= y?=w928:bool)
                        n476 = feedback #44() -> (w933:i64)  [unwired: 1 in]
                        n477 = Add(x=w932, y=w933) -> (x+y=w930:i64)
                        n478 = Select(t=w936, s=w928, f=w927) -> (s? t:f=w937:u32)
                        n479 = feedback-in #43(w937) -> ()
                        n480 = Select(t=i64 0, s=w928, f=w930) -> (s? t:f=w934:i64)
                        n481 = feedback-in #44(w934) -> ()
                        n482 = And(x=w928, y="FPGA Trap Trig") -> (x .and. y?=w935:bool)
                        n483 = case "Trap FB trigger excitation laser ON" shown="True" w935 {
                          tunnel: w930 -> [_ w961]
                          tunnel: w927 -> [_ w959]
                          frame False {
                          }
                          frame True {
                            n484 = Not(x="TTrig Negate Pos") -> (.not. x?=w968:bool)
                            n485 = Boolean To (0,1)(Boolean="TTrig Negate Pos") -> (0, 1=w966:i16)
                            n486 = Boolean To (0,1)(Boolean=w968) -> (0, 1=w967:i16)
                            n487 = Negate(x=w966) -> (-x=w965:i16)
                            n488 = Add(x=w965, y=w967) -> (x+y=w964:i16)
                            n489 = Multiply(x=w964, y=w961) -> (x*y=w963:i64)
                            "TTrig Sig" <- w963
                            n490 = Multiply(x="FPGA TTrig Thresh", y=w959) -> (x*y=w960:i64)
                            "TTrig Fin Thresh" <- w960
                            n491 = Greater Or Equal?(x=w963, y=w960) -> (x >= y?=w962:bool)
                            n492 = case shown="True" w962 {
                              frame False {
                              }
                              frame True {
                                w971 = TRUE ("Green FB On/Off")
                                w973 = u8 2 ("Operating Mode")
                                n493 = local write "Operating Mode 2"(w973) -> ()
                                n494 = local write "Operating Mode"(w973) -> ()
                                n495 = local write "Green FB On/Off"(w971) -> ()
                                n496 = local write "FPGA Trap Trig"(FALSE ("FPGA Trap Trig")) -> ()
                                "TTrig?" <- w971
                              }
                            }
                          }
                        }
                        "Trap Pos FB Int Signal" <- w942
                      }
                    }
                    n497 = feedback-in #42(w907) -> ()
                  }
                }
                n498 = Or(x=w889, y="Start scan") -> (x .or. y?=w881:bool)
                n499 = Not(x="Abort scan") -> (.not. x?=w879:bool)
                n500 = And(x=w879, y=w881) -> (x .and. y?=w878:bool)
                n501 = case "For raster scanning" shown="False" w878 {
                  tunnel: [u64 0 w1042] -> w884
                  tunnel: "Start scan" -> [_ w1027]
                  frame False {
                    n502 = local write "Scanning"(FALSE ("scanning")) -> ()
                  }
                  frame True {
                    w1011 = i64 0
                    w1010 = u64 0
                    # "scan incr."
                    # "freq. incr. mult."
                    # "count steps"
                    # "count number of cycles"
                    n503 = feedback #45(w1010) -> (w1039:u64)
                    n504 = Select(t=w1010, s=w1027, f=w1039) -> (s? t:f=w1041:u64)
                    n505 = Increment(x=w1041) -> (x+1=w1038:u64)
                    n506 = Greater?(x="Cycles per step", y=w1038) -> (0:w1020:bool)
                    n507 = Select(t=w1038, s=w1020, f=w1010) -> (s? t:f=w1037:u64)
                    n508 = feedback-in #45(w1037) -> ()
                    n509 = feedback #46(w1010) -> (w1036:u64)
                    n510 = Select(t=w1010, s=w1027, f=w1036) -> (s? t:f=w1031:u64)
                    n511 = Increment(x=w1031) -> (x+1=w1035:u64)
                    n512 = Add(x="Scan steps", y="Scan steps") -> (x+y=w1034:u64)
                    n513 = Select(t=w1031, s=w1020, f=w1035) -> (s? t:f=w1015:u64)
                    n514 = Greater?(x=w1034, y=w1015) -> (0:w1014:bool)
                    n515 = Select(t=w1015, s=w1014, f=w1010) -> (s? t:f=w1032:u64)
                    n516 = feedback-in #46(w1032) -> ()
                    n517 = Equal?(x="Scan steps", y=w1015) -> (x = y?=w1019:bool)
                    n518 = Greater?(x="Scan steps", y=w1031) -> (0:w1030:bool)
                    n519 = feedback #47(w1011) -> (w1033:i64)
                    n520 = Select(t=w1011, s=w1027, f=w1033) -> (s? t:f=w1017:i64)
                    n521 = Increment(x=w1017) -> (x+1=w1029:i64)
                    n522 = Decrement(x=w1017) -> (x-1=w1028:i64)
                    n523 = Select(t=w1029, s=w1030, f=w1028) -> (s? t:f=w1018:i64)
                    n524 = Select(t=w1017, s=w1019, f=w1018) -> (s? t:f=w1016:i64)
                    n525 = Select(t=w1017, s=w1020, f=w1016) -> (s? t:f=w1012:i64)
                    n526 = Select(t=w1012, s=w1014, f=w1011) -> (s? t:f=w1013:i64)
                    n527 = feedback-in #47(w1013) -> ()
                    n528 = feedback #48(w1010) -> (w1026:u64)
                    n529 = Select(t=w1010, s=w1027, f=w1026) -> (s? t:f=w1022:u64)
                    n530 = Increment(x=w1022) -> (x+1=w1023:u64)
                    n531 = Select(t=w1022, s=w1014, f=w1023) -> (s? t:f=w1021:u64)
                    n532 = Greater?(x="Number of scans", y=w1021) -> (0:w1007:bool)
                    n533 = Multiply(x="Scan freq.  increment", y=w1017) -> (x*y=w1042:i64)
                    n534 = Select(t=TRUE, s="Cont. Scan", f=w1007) -> (s? t:f=w1006:bool)
                    "Scanning" <- w1006
                    n535 = Select(t=w1021, s=w1006, f=w1010) -> (s? t:f=w1024:u64)
                    n536 = feedback-in #48(w1024) -> ()
                    n537 = Increment(x=w1021) -> (x+1=→"Scan I":u64)
                  }
                }
                n538 = case "For intensity feedback" shown="True" "FB On/Off Set 1" {
                  tunnel: "BD 1 Amplitude 1" -> [w1044 _]
                  tunnel: [w1044 w1045] -> w876
                  frame False {
                  }
                  frame True {
                    n539 = local read "AI2 Y Sum Set 1"() -> (w1047:i16)
                    n540 = call "Slower PID.vi"("process variable"=w1047, "reset?"="FB Reset Set 1", "setpoint"="FB Setpoint Set 1", "PID gains (x 2^8)"="FB Gains Set 1", "output range"="FB output range 1") -> ("output"=w1050:i16)  [unwired: 10 out]
                    n541 = To Unsigned Word Integer(number=w1050) -> (unsigned 16bit integer=w1045:u16)
                  }
                }
                n542 = Select(t=w883, s="Scan BD", f=w884) -> (s? t:f=w882:u64)
                n543 = Select(t=w884, s="Scan BD", f=w883) -> (s? t:f=w885:u64)
                n544 = Add(x=w882, y="BD 2 Frequency 1") -> (x+y=w887:u64)
                n545 = Compound Arithmetic op=ADD("BD 1 Frequency 1", w873, w885) -> (w888:u64)
                "BD1 Frequency Out 1" <- w888
              }
              frame 2 {
                # "Trap 2"
                n546 = case shown="True" "FB On/Off Set 2" {
                  tunnel: [w1058 w1059] -> w1054
                  tunnel: "BD 1 Amplitude 2" -> [w1058 _]
                  frame False {
                  }
                  frame True {
                    n547 = local read "AI2 Y Sum Set 2"() -> (w1064:i16)
                    n548 = call "Slower PID.vi"("process variable"=w1064, "reset?"="FB Reset Set 2", "setpoint"="FB Setpoint Set 2", "PID gains (x 2^8)"="FB Gains Set 2", "output range"="FB output range 2") -> ("output"=w1061:i16)  [unwired: 10 out]
                    n549 = To Unsigned Word Integer(number=w1061) -> (unsigned 16bit integer=w1059:u16)
                  }
                }
                "BD1 Frequency Out 2" <- "BD 1 Frequency 2"
              }
              frame 3 {
                # "Fluorescence period"
              }
            }
            n550 = feedback-in #49(w790) -> ()
            n551 = feedback #49(w790) -> (w789:u32)
            n552 = Select(t=w792, s="Interlace ON/OFF", f="Interlace Off Parameters") -> (s? t:f=w830:u8)
            n553 = Subtract(x=w790, y=w789) -> (x-y=w788:u32)
            n554 = Subtract "The error"(x=w788, y=w787) -> (x-y=w765:u32)
            n555 = case shown="1, Default" w830 {
              tunnel: ["DIO count 1 (ticks)" "DIO count 2 (ticks)" "DIO count 3 (ticks)"] -> w786
              frame 1, Default {
              }
              frame 2 {
              }
              frame 3 {
              }
            }
            n556 = Number To Boolean Array(number=w765) -> (Boolean array=w766:bool[])
            n557 = Or Array Elements(Boolean array=w766) -> (logical OR=w764:bool)
            "DIO Late?" <- w764
            n558 = Boolean To (0,1)(Boolean=w764) -> (0, 1=w771:i16)
            n559 = To Unsigned Word Integer(number=w771) -> (unsigned 16bit integer=w768:u16)
            n560 = feedback #50(u16 0) -> (w769:u16)
            n561 = Add(x=w768, y=w769) -> (x+y=w767:u16)
            "DIO Late Counter" <- w767
            n562 = feedback-in #50(w767) -> ()
            n563 = Subtract(x=w786, y=w765) -> (x-y=w785:u32)
            n564 = Split Number(x=w827) -> (hi(x)=w826:u32, lo(x)=w825:u32)
            n565 = Split Number(x=w816) -> (hi(x)=w821:u32, lo(x)=w820:u32)
            n566 = Boolean To (0,1)(Boolean="+ phase (DIO)") -> (0, 1=w782:i16)
            n567 = Split Number(x=w826) -> (lo(x)=w824:u16)  [unwired: 1 out]
            n568 = Split Number(x=w825) -> (hi(x)=w823:u16, lo(x)=w822:u16)
            n569 = Split Number(x=w821) -> (lo(x)=w819:u16)  [unwired: 1 out]
            n570 = Split Number(x=w820) -> (hi(x)=w818:u16, lo(x)=w817:u16)
            n571 = Split Number(x=w775) -> (hi(x)=w777:u8, lo(x)=w776:u8)
            n572 = Split Number(x=w772) -> (hi(x)=w774:u8, lo(x)=w773:u8)
            n573 = Split Number(x=w824) -> (hi(x)=w814:u8, lo(x)=w813:u8)
            n574 = Split Number(x=w823) -> (hi(x)=w812:u8, lo(x)=w811:u8)
            n575 = Split Number(x=w819) -> (hi(x)=w807:u8, lo(x)=w806:u8)
            n576 = Split Number(x=w822) -> (hi(x)=w810:u8, lo(x)=w809:u8)
            n577 = Split Number(x=w818) -> (hi(x)=w805:u8, lo(x)=w804:u8)
            n578 = Split Number(x=w817) -> (hi(x)=w803:u8, lo(x)=w802:u8)
            n579 = Multiply(x=w782, y="Phase count adjustment (DIO)") -> (x*y=w778:i16)
            n580 = feedback #51(i16 0) -> (w780:i16)
            n581 = Subtract(x=w780, y=w778) -> (x-y=w779:i16)
            "DIO Relative phase" <- w779
            n582 = feedback-in #51(w779) -> ()
            n583 = Add(x=w785, y=w778) -> (x+y=w784:u32)
            n584 = Build Array "BD 1 A Stack"(w777, w776) -> (w799:u8[])
            n585 = Build Array "BD 2 A Stack"(w774, w773) -> (w798:u8[])
            n586 = Build Array "BD 1 nu Stack"(w814, w813, w812, w811, w810, w809) -> (w808:u8[])
            n587 = Build Array "BD 2 nu Stack"(w807, w806, w805, w804, w803, w802) -> (w801:u8[])
            n588 = case shown="2" w815 {
              tunnel: [w865 w868] -> w797
              tunnel: [u8 10 u8 4] -> w800
              tunnel: "Swap F1 and F2" -> [w866 w868]
              frame 2 {
                # "F2"
                n589 = Not(x=w866) -> (.not. x?=w865:bool)
              }
              frame 1, Default {
                # "low chooses F1"
                # "F1"
              }
            }
            n590 = case "If FPGA is controlling (toggling) RF synth" shown="True" w796 {
              tunnel: w808 -> [_ w844]
              tunnel: w801 -> [_ w843]
              tunnel: w800 -> [_ w842]
              tunnel: w799 -> [_ w841]
              tunnel: w798 -> [_ w840]
              frame False {
              }
              frame True {
                # "Write next amp.\n(wait until beginning of next loop iteration to update)"
                n591 = flat-sequence "Update the next F1 and F2 frequency value (the actual frequency won't change until FSK is switched).\nThen load the next amplitude value into buffer, but don't update it until the next cycle." {
                  tunnel: w844 -> [w847]
                  tunnel: w843 -> [w846]
                  tunnel: w842 -> [w845]
                  tunnel: w841 -> [w858]
                  tunnel: w840 -> [w857]
                  frame #0 {
                    n592 = for {
                      tunnel: w847 -> [w853] mode=indexing
                      tunnel: w846 -> [w852] mode=indexing
                      tunnel: w845 -> [w850]
                      i -> [w851]
                      # "Write next freq."
                      n593 = To Unsigned Byte Integer(number=w851) -> (unsigned 8bit integer=w848:u8)
                      n594 = Add(x=w850, y=w848) -> (x+y=w849:u8)
                      n595 = call "write to RF synth bd.vi"("Address Byte"=w849, "BD 2 Byte"=w852, "BD 1 Byte"=w853) -> ()
                    }
                  }
                  frame #1 {
                    # "send udclk high"
                    n596 = xnode "FPGA I/O Node"("Connector1/DIO30"=TRUE ("Connector1/DIO15")) -> ()  [unwired: 1 in, 1 out]
                  }
                  frame #2 {
                    n597 = xnode "FPGA I/O Node"("Connector1/DIO30"=FALSE ("Connector1/DIO15")) -> ()  [unwired: 1 in, 1 out]
                  }
                  frame #3 {
                    n598 = for {
                      tunnel: w858 -> [w864] mode=indexing
                      tunnel: w857 -> [w863] mode=indexing
                      tunnel: u8 33 -> [w861]
                      i -> [w862]
                      n599 = To Unsigned Byte Integer(number=w862) -> (unsigned 8bit integer=w859:u8)
                      n600 = Add(x=w861, y=w859) -> (x+y=w860:u8)
                      n601 = call "write to RF synth bd.vi"("Address Byte"=w860, "BD 2 Byte"=w863, "BD 1 Byte"=w864) -> ()
                    }
                  }
                }
              }
            }
          }
        }
      }
    }
  }
  n602 = node-c288(w4) -> ()
